vi "Emballage_BDD_motDePasse_remplacerValve.vi"() -> (2 "Booléen":bool)   [LabVIEW 2020]
panel:
  out "Tableau 2":bool[][](array[boolean])
  out "Numérique":i32
  in  "A 2":bool
  in  "A 3":bool
  in  "A 6":bool
  in  "A 5":bool
  in  "A 4":bool
  in  "A 1":bool
  in  "A 8":bool
  in  "A 7":bool
  in  "A 9":bool
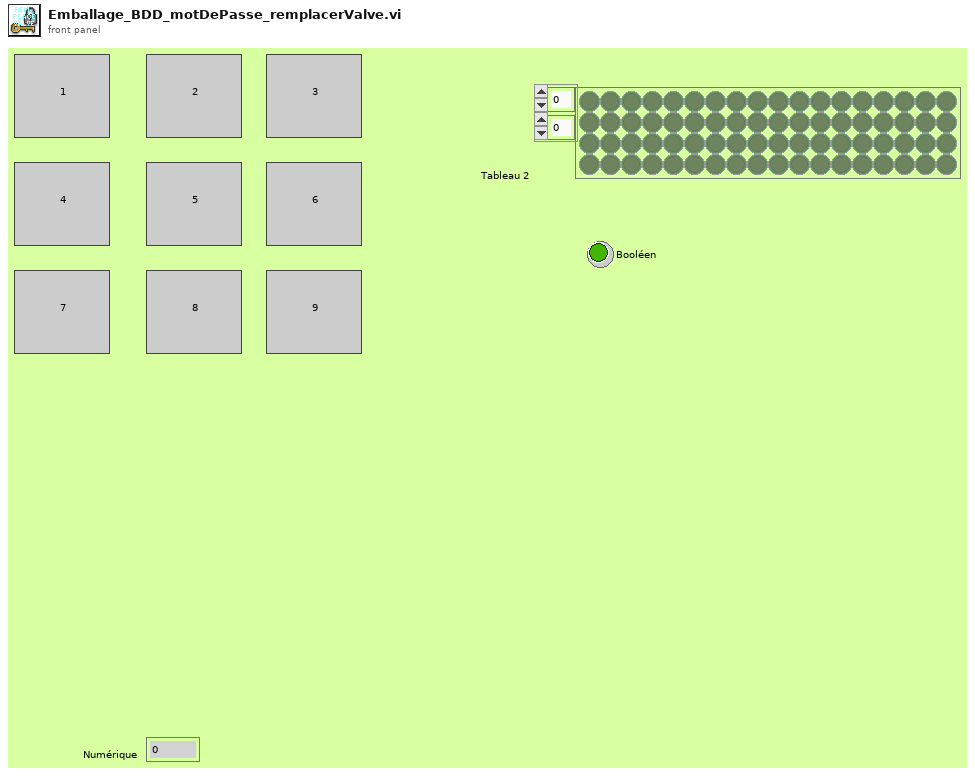
[diagram p1: front panel]
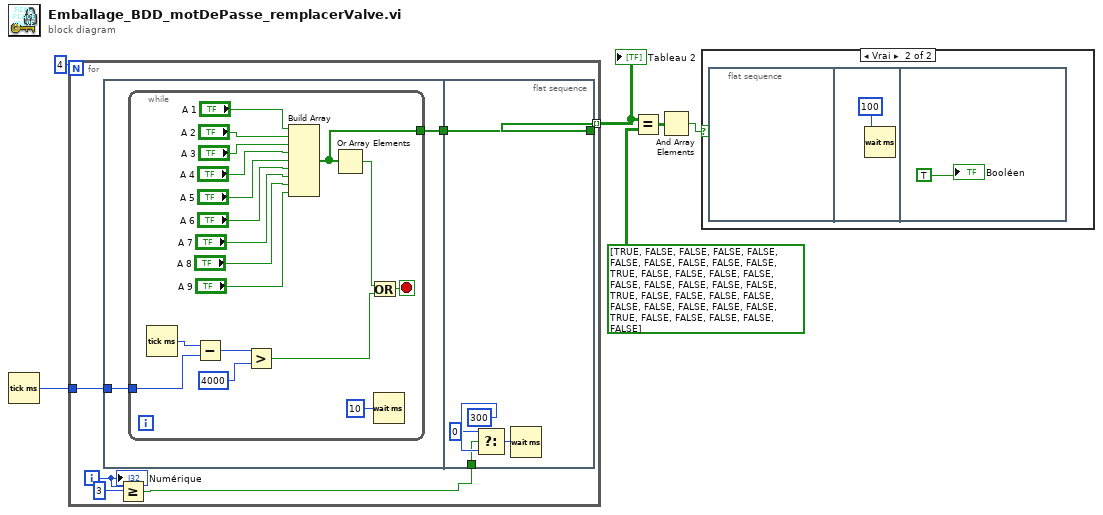
[diagram p0: block diagram]
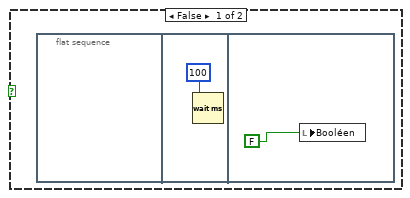
[diagram p2: hidden frame]
diagram:
  n1 = Tick Count (ms)() -> (millisecond timer value=w1:u32)
  n2 = for {
    N: 4 -> [_]
    tunnel: [w12] -> w3 mode=indexing
    tunnel: w1 -> [w7]
    i -> [w10]
    n3 = flat-sequence {
      tunnel: [w14] -> w11
      tunnel: w7 -> [w13]
      tunnel: [w37] -> w12
      tunnel: w11 -> [w37]
      tunnel: w8 -> [w35]
      frame #0 {
        n4 = while {
          tunnel: [w22] -> w14
          tunnel: w13 -> [w18]
          stop <- w20 stop-if-true
          n5 = Tick Count (ms)() -> (millisecond timer value=w19:u32)
          n6 = Subtract(x=w19, y=w18) -> (x-y=w17:u32)
          n7 = Greater?(x=w17, y=u32 4000) -> (0:w15:bool)
          n8 = Build Array("A 1", "A 2", "A 3", "A 4", "A 5", "A 6", "A 7", "A 8", "A 9") -> (w22:bool[])
          n9 = Or Array Elements(Boolean array=w22) -> (logical OR=w23:bool)
          n10 = Or(x=w23, y=w15) -> (x .or. y?=w20:bool)
          n11 = Wait (ms)(milliseconds to wait=u32 10 ("attente (ms)")) -> ()  [unwired: 1 out]
        }
      }
      frame #1 {
        n12 = Select(t=u32 0 ("cas vrai"), s=w35, f=u32 300 ("attente (ms)")) -> (s? t:f=w33:u32)
        n13 = Wait (ms)(milliseconds to wait=w33) -> ()  [unwired: 1 out]
      }
    }
    n14 = Greater Or Equal?(x=w10, y=3) -> (x >= y?=w8:bool)
    "Numérique" <- w10
  }
  "Tableau 2" <- w3
  n15 = Equal?(x=w3, y=bool[][] [[TRUE, FALSE, FALSE, FALSE, FALSE, FALSE, FALSE, FALSE, FALSE], [FALSE, TRUE, FALSE, FALSE, FALSE, FALSE, FALSE, FALSE, FALSE], [FALSE, FALSE, TRUE, FALSE, FALSE, FALSE, FALSE, FALSE, FALSE], [FALSE, FALSE, FALSE, TRUE, FALSE, FALSE, FALSE, FALSE, FALSE]]) -> (x = y?=w5:bool[][])
  n16 = And Array Elements(Boolean array=w5) -> (logical AND=w6:bool)
  n17 = case shown="Vrai" w6 {
    frame False {
      n18 = flat-sequence {
        frame #0 {
        }
        frame #1 {
          n19 = Wait (ms)(milliseconds to wait=u32 100 ("attente (ms)")) -> ()  [unwired: 1 out]
        }
        frame #2 {
          n20 = local write "Booléen"(FALSE ("Visible")) -> ()
        }
      }
    }
    frame True {
      n21 = flat-sequence {
        frame #0 {
        }
        frame #1 {
          n22 = Wait (ms)(milliseconds to wait=u32 100 ("attente (ms)")) -> ()  [unwired: 1 out]
        }
        frame #2 {
          "Booléen" <- TRUE ("Visible")
        }
      }
    }
  }
